vi "niTuner Config Scan Advance.vi"(4 "ready signal parameters":T1={"type"=enum."pulse", "polarity"=enum."active low", "pulse length (sec)"=1e-06} {"pulse length (sec)" format="%.2p"}, 6 "advance signal parameters":T2, 8 "error in":errorcluster, 9 "ready signal":T3(ring)=enum."no change", 10 "advance trigger":T4(ring)=enum."no change", 11 "taskID in":i32 format="%.0x") -> (0 "error out":errorcluster, 3 "taskID out":i32 format="%.0x")   [LabVIEW 2011]
doc: "This VI configures the scan advance trigger input and the ready signal output. The advance trigger tells the PXI-5600 downconverter to advance to the next frequency in the scan list. The ready signal is generated after the downconverter has settled to a frequency."
uses:
  nipxi5600u.dll
panel:
  # "OPTIONAL:"
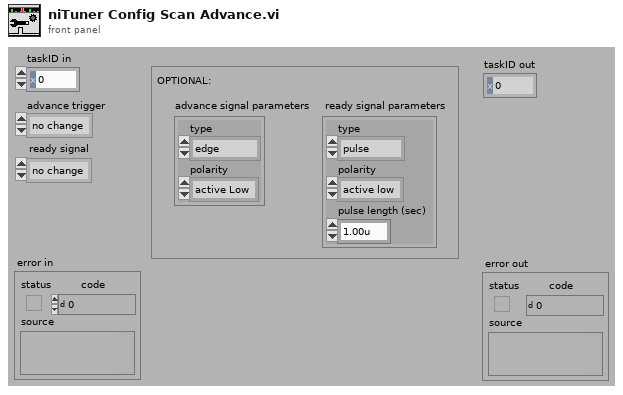
[diagram p1: front panel]
types:
  T1 = cluster{"type":enum32{"pulse", "level"}, "polarity":enum32{"active low", "active high"}, "pulse length (sec)":dbl}
  T2 = cluster{"type":enum32{"edge", "level"}, "polarity":enum32{"active Low", "active high"}}
  T3 = enum32{"none", "RTSI 0", "RTSI 1", "RTSI 2", "RTSI 3", "RTSI 4", "RTSI 5", "RTSI 6", "no change"}
  T4 = enum32{"software", "RTSI 0", "RTSI 1", "RTSI 2", "RTSI 3", "RTSI 4", "RTSI 5", "RTSI 6", "no change"}
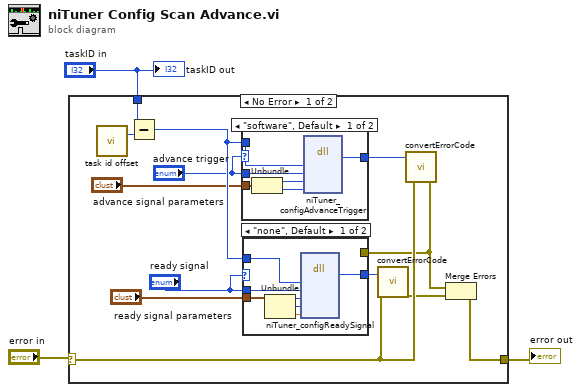
[diagram p0: block diagram]
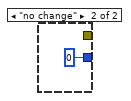
[diagram p2: hidden frame]
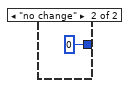
[diagram p3: hidden frame]
diagram:
  n1 = case shown="No Error" "error in" {
    selector: "error in" -> [w11 w32]
    tunnel: [w9 w32] -> w2
    tunnel: "taskID in" -> [w14 _]
    frame No Error {
      n2 = call <instrlib>:"task id offset.vi"() -> ("taskID offset"=w15:i32)
      n3 = Subtract(x=w14, y=w15) -> (x-y=w13:i32)
      n4 = case shown="\"software\", Default" "advance trigger" {
        tunnel: [w30 0] -> w16
        tunnel: "advance trigger" -> [w29 _]
        tunnel: w13 -> [w28 _]
        tunnel: "advance signal parameters" -> [w27 _]
        frame "software", Default {
          n5 = Unbundle(w27) -> ("type"=w26:enum32{"edge", "level"}, "polarity"=w25:enum32{"active Low", "active high"})
          n6 = dll-call lib="nipxi5600u.dll" fn="niTuner_configAdvanceTrigger"("taskID"=w28, "advanceTriggerSource"=w29, "advanceType"=w26, "advancePolarity"=w25) -> (w30:i32)  [unwired: 7 in, 2 out]
        }
        frame "no change" {
        }
      }
      n7 = call <instrlib>:"convertErrorCode.vi"("error in"=w11, "error code"=w16) -> ("error out"=w4:errorcluster)
      n8 = case shown="\"none\", Default" "ready signal" {
        tunnel: w13 -> [w23 _]
        tunnel: [w22 0] -> w12
        tunnel: "ready signal" -> [w21 _]
        tunnel: "ready signal parameters" -> [w20 _]
        tunnel: w4 -> [_ _]
        frame "none", Default {
          n9 = Unbundle(w20) -> ("type"=w19:enum32{"pulse", "level"}, "polarity"=w18:enum32{"active low", "active high"}, "pulse length (sec)"=w17:dbl)
          n10 = dll-call lib="nipxi5600u.dll" fn="niTuner_configReadySignal"("taskID"=w23, "readyDestination"=w21, "readyType"=w19, "readyPolarity"=w18, "pulseLength"=w17) -> (w22:i32)  [unwired: 8 in, 2 out]
        }
        frame "no change" {
        }
      }
      n11 = call <instrlib>:"convertErrorCode.vi"("error in"=w11, "error code"=w12) -> ("error out"=w10:errorcluster)
      n12 = Merge Errors(w4, w10) -> (w9:errorcluster)
    }
    frame Error {
    }
  }
  "error out" <- w2
  "taskID out" <- "taskID in"
